vi "Read.vi"(8 "error in (no error)":errorcluster, 11 "Behavior in":refnum<class "BehaviorData.lvclass">) -> (0 "error out":errorcluster, 3 "Behavior out":refnum<class "BehaviorData.lvclass">)   [LabVIEW 2010, in "BehaviorData.lvclass"]
uses:
  BehaviorData.lvclass
  BehaviorData.lvclass/BehaviorData.ctl
panel:
  out "Backlog":u32
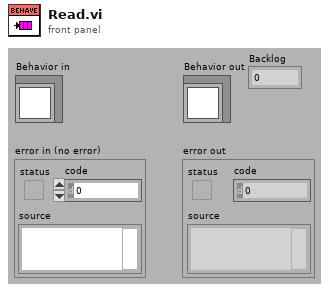
[diagram p1: front panel]
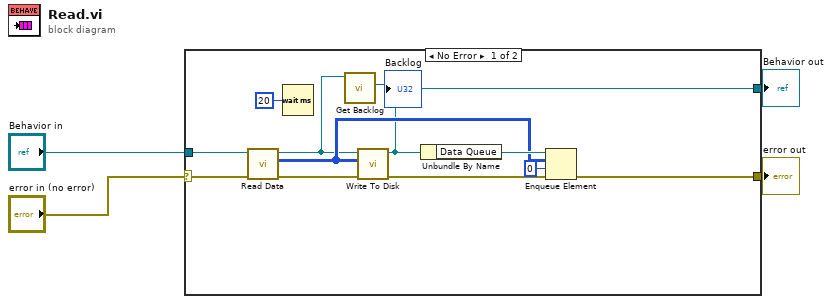
[diagram p0: block diagram]
diagram:
  n1 = case shown="No Error" "error in (no error)" {
    selector: "error in (no error)" -> [w15 w18]
    tunnel: [w9 w18] -> w3
    tunnel: [w5 w17] -> w1
    tunnel: "Behavior in" -> [w14 w17]
    frame No Error {
      n2 = call-dynamic "Read Data.vi"("error in (no error)"=w15, "AcquireTraces in"=w14) -> ("error out"=w13:errorcluster, "data"=w10:i32[][], "AcquireTraces out"=w8:refnum<class "BehaviorData.lvclass">)  [unwired: 7 in]
      n3 = Wait (ms)(milliseconds to wait=u32 20) -> ()  [unwired: 1 out]
      n4 = call-dynamic "Get Backlog.vi"("AcquireTraces in"=w8) -> ("Backlog"=→"Backlog":u32)  [unwired: 8 in, 2 out]
      n5 = call-dynamic "Write To Disk.vi"("error in (no error)"=w13, "element"=w10, "AcquireTraces in"=w8) -> ("error out"=w11:errorcluster, "AcquireTraces out"=w5:refnum<class "BehaviorData.lvclass">)  [unwired: 7 in]
      n6 = Unbundle By Name(w5) -> ("Data Queue"=w12:refnum<queue>)
      n7 = Enqueue Element(queue=w12, element=w10, timeout in ms (-1)=0, error in (no error)=w11) -> (error out=w9:errorcluster)  [unwired: 2 out]
    }
    frame Error {
    }
  }
  "error out" <- w3
  "Behavior out" <- w1
